vi "Get Data Length.vi"(11 "variant in":variant) -> (1 "number of samples":i32, 3 "variant out":variant)   [LabVIEW 2017]
uses:
  <vilib>/addons/_NISVFA/_Shared subVIs/Controls/NI Channel Properties.ctl
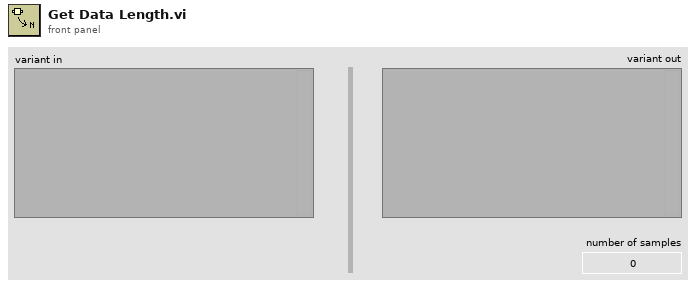
[diagram p1: front panel]
types:
  T1 = typedef "NI Channel Properties.ctl" = u16
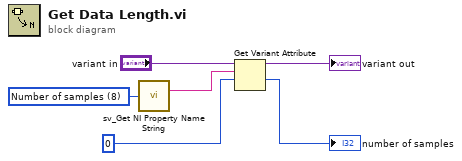
[diagram p0: block diagram]
diagram:
  w2 = T1 8 items=["Channel name", "Channel description", "Axis label", "Unit string", "Waveform X-axis label", "Waveform X-axis unit string", "x0", "dx", "Number of samples", "X channel", "Filter settled", "dB reference", "Window", "Window parameter", "Window size", "FFT size", "Peak units", "Spectrum type", "Magnitude scale", "Spectral density", "Sensor sensitivity (mV/EU)", "X-axis dimension", "LabVIEW datatype", "Function type", "Function subtype", "X values", "Independent channel", "Column index", "Collection name", "Collection ID", "X Columns", "Phase unwrapped"] ("property")
  n1 = call <vilib>:"sv_Get NI Property Name String.vi"("property"=w2) -> ("TDMS property name"=w1:string)  [unwired: 13 in, 1 out]
  n2 = Get Variant Attribute(Variant="variant in", name=w1, default value (empty Variant)=0 ("timestamp")) -> (duplicate Variant=→"variant out":variant, value=→"number of samples":i32)  [unwired: 1 in, 2 out]
